vi "Send Acyclic Frames.vi"(8 "error in":errorcluster, 10 "transfer ids":u16[](array[numeric]), 11 "module handle":u32) -> (0 "error out":errorcluster, 3 "module handle out":u32)   [LabVIEW 2020, in "AIM MIL-STD-1553 Hardware API.lvlib"]
uses:
  AIM MIL-STD-1553 Hardware API.lvlib
  Global - Disable Hardware API Constant.vi
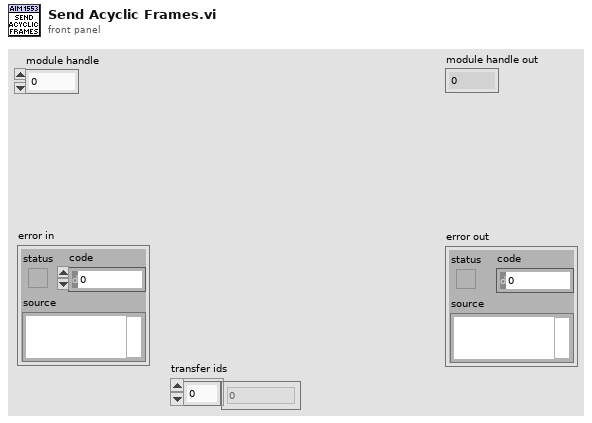
[diagram p1: front panel]
types:
  T1 = enum16{"Enabled (Default)", "Disabled for Unit Testing"}
  T2 = enum16{"API_BC_ACYC_SEND_IMMEDIATELY", "API_BC_ACYC_SEND_ON_TIMETAG", "API_BC_ACYC_SEND_AT_END_OF_FRAME"}
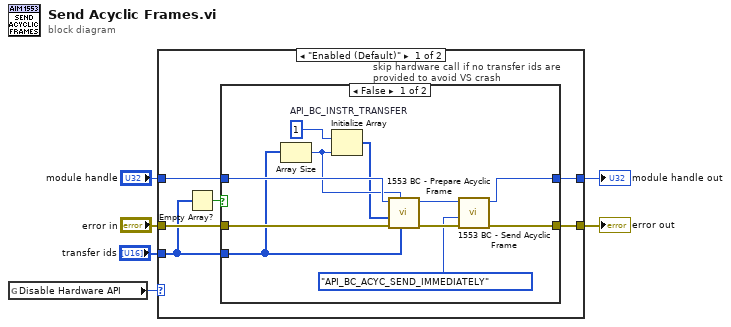
[diagram p0: block diagram]
diagram:
  n1 = global read "Global - Disable Hardware API Constant.vi" "Disable Hardware API"() -> (w1:T1)
  n2 = case shown="\"Enabled (Default)\"" w1 {
    tunnel: [w12 w26] -> w6
    tunnel: "error in" -> [w11 w26]
    tunnel: "transfer ids" -> [w7 _]
    tunnel: "module handle" -> [w10 w27]
    tunnel: [w9 w27] -> w2
    frame "Enabled (Default)" {
      n3 = Empty Array?(array=w7) -> (empty?=w8:bool)
      n4 = case "skip hardware call if no transfer ids are provided to avoid VS crash" shown="False" w8 {
        tunnel: [w23 w24] -> w12
        tunnel: w11 -> [w21 w24]
        tunnel: w10 -> [w20 w25]
        tunnel: [w17 w25] -> w9
        tunnel: w7 -> [w16 _]
        frame False {
          w14 = 1  # API_BC_INSTR_TRANSFER
          n5 = Array Size(array=w16) -> (size(s)=w15:i32)
          n6 = Initialize Array(w14, w15) -> (w13:i32[])
          n7 = call <instrlib>:"1553 BC - Prepare Acyclic Frame.vi"("Xid"=w16, "Cnt"=w15, "Error In (none)"=w21, "Instruction"=w13, "Module Handle"=w20) -> ("Error Out"=w22:errorcluster, "Module Handle Out"=w19:u32)  [unwired: 5 in]
          n8 = call <instrlib>:"1553 BC - Send Acyclic Frame.vi"("Error In (none)"=w22, "Mode"=T2."API_BC_ACYC_SEND_IMMEDIATELY", "Module Handle"=w19) -> ("Error Out"=w23:errorcluster, "Module Handle Out"=w17:u32)  [unwired: 7 in]
        }
        frame True {
        }
      }
    }
    frame "Disabled for Unit Testing" {
    }
  }
  "error out" <- w6
  "module handle out" <- w2
